vi "Generator de semnale multiple folosind module de tipuri diferite.vi"() -> ()   [LabVIEW 2011]
uses:
  <vilib>/measure/NI_MABase.lvlib
panel:
  in  "Signal Source":T1(ring)
  in  "stop":bool
  in  "Square duty cycle (%)":dbl
  in  "Phase":dbl
  in  "Amplitude":dbl
  in  "Frequency":dbl
  in  "Sampling 0":cluster{"Fs":dbl, "#s":dbl}
  out "error out":errorcluster
  out "Waveform Graph":waveform(dbl)(graph)
  in  "Reset phase":bool
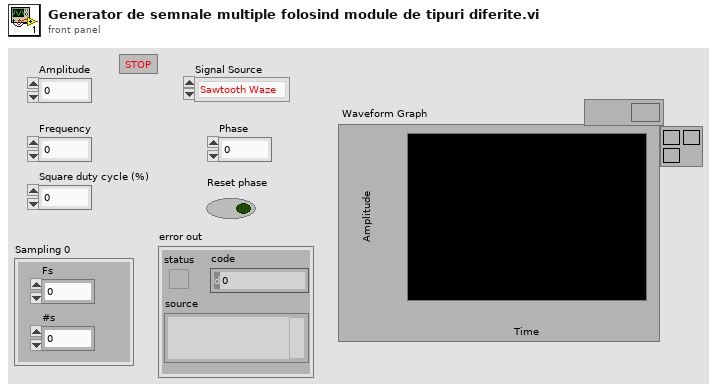
[diagram p1: front panel]
types:
  T1 = enum16{"Sawtooth Waze", "Square Waze\n", "Triangle Waze"}
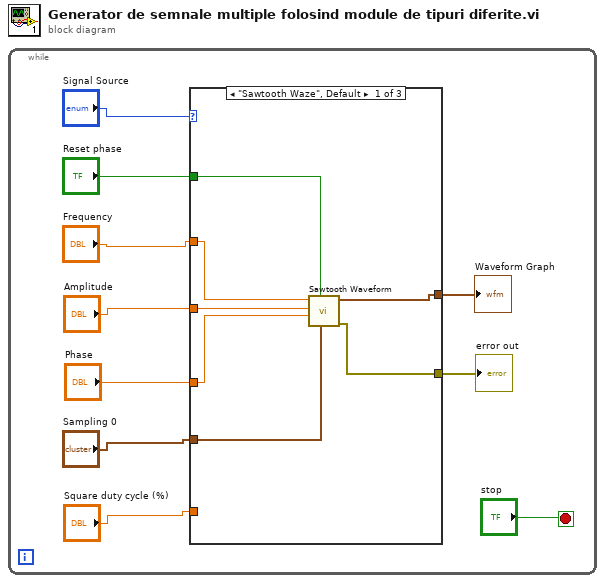
[diagram p0: block diagram]
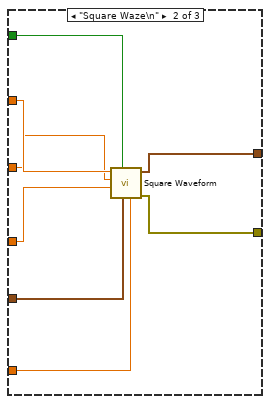
[diagram p2: hidden frame]
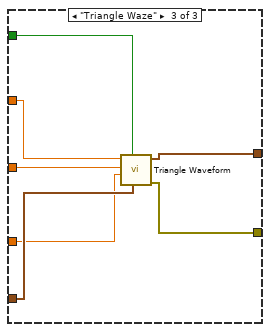
[diagram p3: hidden frame]
diagram:
  n1 = while {
    stop <- "stop" stop-if-true
    n2 = case shown="\"Sawtooth Waze\", Default" "Signal Source" {
      tunnel: "Reset phase" -> [w17 w25 w26]
      tunnel: "Frequency" -> [w16 w24 w27]
      tunnel: "Amplitude" -> [w15 w23 w28]
      tunnel: "Phase" -> [w14 w22 w29]
      tunnel: "Sampling 0" -> [w13 w21 w30]
      tunnel: "Square duty cycle (%)" -> [_ w20 _]
      tunnel: [w12 w18 w32] -> w2
      tunnel: [w11 w19 w31] -> w1
      frame "Sawtooth Waze", Default {
        n3 = call <vilib>:"Sawtooth Waveform.vi"("sampling info"=w13, "reset signal"=w17, "phase"=w14, "amplitude"=w15, "frequency"=w16) -> ("error out"=w11:errorcluster, "signal out"=w12:waveform(dbl))  [unwired: 5 in]
      }
      frame "Square Waze\n" {
        n4 = call <vilib>:"Square Waveform.vi"("duty cycle (%)"=w20, "sampling info"=w21, "reset signal"=w25, "phase"=w22, "amplitude"=w23, "frequency"=w24) -> ("error out"=w19:errorcluster, "signal out"=w18:waveform(dbl))  [unwired: 4 in]
      }
      frame "Triangle Waze" {
        n5 = call <vilib>:"Triangle Waveform.vi"("sampling info"=w30, "reset signal"=w26, "phase"=w29, "amplitude"=w28, "frequency"=w27) -> ("error out"=w31:errorcluster, "signal out"=w32:waveform(dbl))  [unwired: 5 in]
      }
    }
    "Waveform Graph" <- w2
    "error out" <- w1
  }
